vi "GTCP331-200ER - 1.C.(4).vi"(8 "error in (no error)":errorcluster, 11 "RT - Analysis Data in in in":T1={"Accel Sensistivity"=[0.0, 0.0, 0.0], "Cutoff Frequncies"=[{"LP Passband"=0.0, "HP Stopband"=0.0, "LP Stopband"=0.0, "HP Passband"=0.0}, {"LP Passband"=0.0, "HP Stopband"=0.0, "LP Stopband"=0.0, "HP Passband"=0.0}, {"LP Passband"=0.0, "HP Stopband"=0.0, "LP Stopband"=0.0, "HP Passband"=0.0}], "APU Setup File"={"Sensor Info"=[], "Calibration Info"=[], "CMM Table 106"=[], "CMM Table 106B "=[], "Accel Config"=[], "Report Sheet 1"=[], "Report Sheet 2"=[], "Report Sheet 3"=[]}, "RepairLevel"=""} {"Cutoff Frequncies"."HP Passband" min=1.0 step=1.0 format="%#.4f"; "Cutoff Frequncies"."LP Stopband" min=1.0 step=1.0 format="%#.4f"; "Cutoff Frequncies"."HP Stopband" min=1.0 step=1.0 format="%#.4f"; "Cutoff Frequncies"."LP Passband" min=1.0 step=1.0 format="%#.4f"}) -> (0 "error out":errorcluster, 2 "Interactive Mode Vals":dbl[](array[numeric]), 3 "RT - Analysis Data in out":T1 {"Cutoff Frequncies"."HP Passband" min=1.0 step=1.0 format="%#.4f"; "Cutoff Frequncies"."LP Stopband" min=1.0 step=1.0 format="%#.4f"; "Cutoff Frequncies"."HP Stopband" min=1.0 step=1.0 format="%#.4f"; "Cutoff Frequncies"."LP Passband" min=1.0 step=1.0 format="%#.4f"})   [LabVIEW 2018, in "RT - Analysis.lvlib"]
doc: "This subtest perfmors engine run-in procedures."
uses:
  RT - Analysis.lvlib
  Private Controls/Watchdog Settings.ctl
  Private Controls/Interactive Data.ctl
  <vilib>/Analysis/NI_AALBase.lvlib
  <vilib>/Analysis/baseanly.llb/Mean (DBL).vi
  Private Controls/RT-Analysis Data.ctl
  Modules/Testing UI 3/Private Controls/Cutoff Frequency.ctl
  Modules/Testing UI 3/Testing UI 3.lvlib
  Top Level/Shared Controls/APU Setup File.ctl
panel:
  # "Highpass Cutoff Frequency"
  # "Lowpass Cutoff Frequency"
  # "Highpass Cutoff Frequency"
  # "Lowpass Cutoff Frequency"
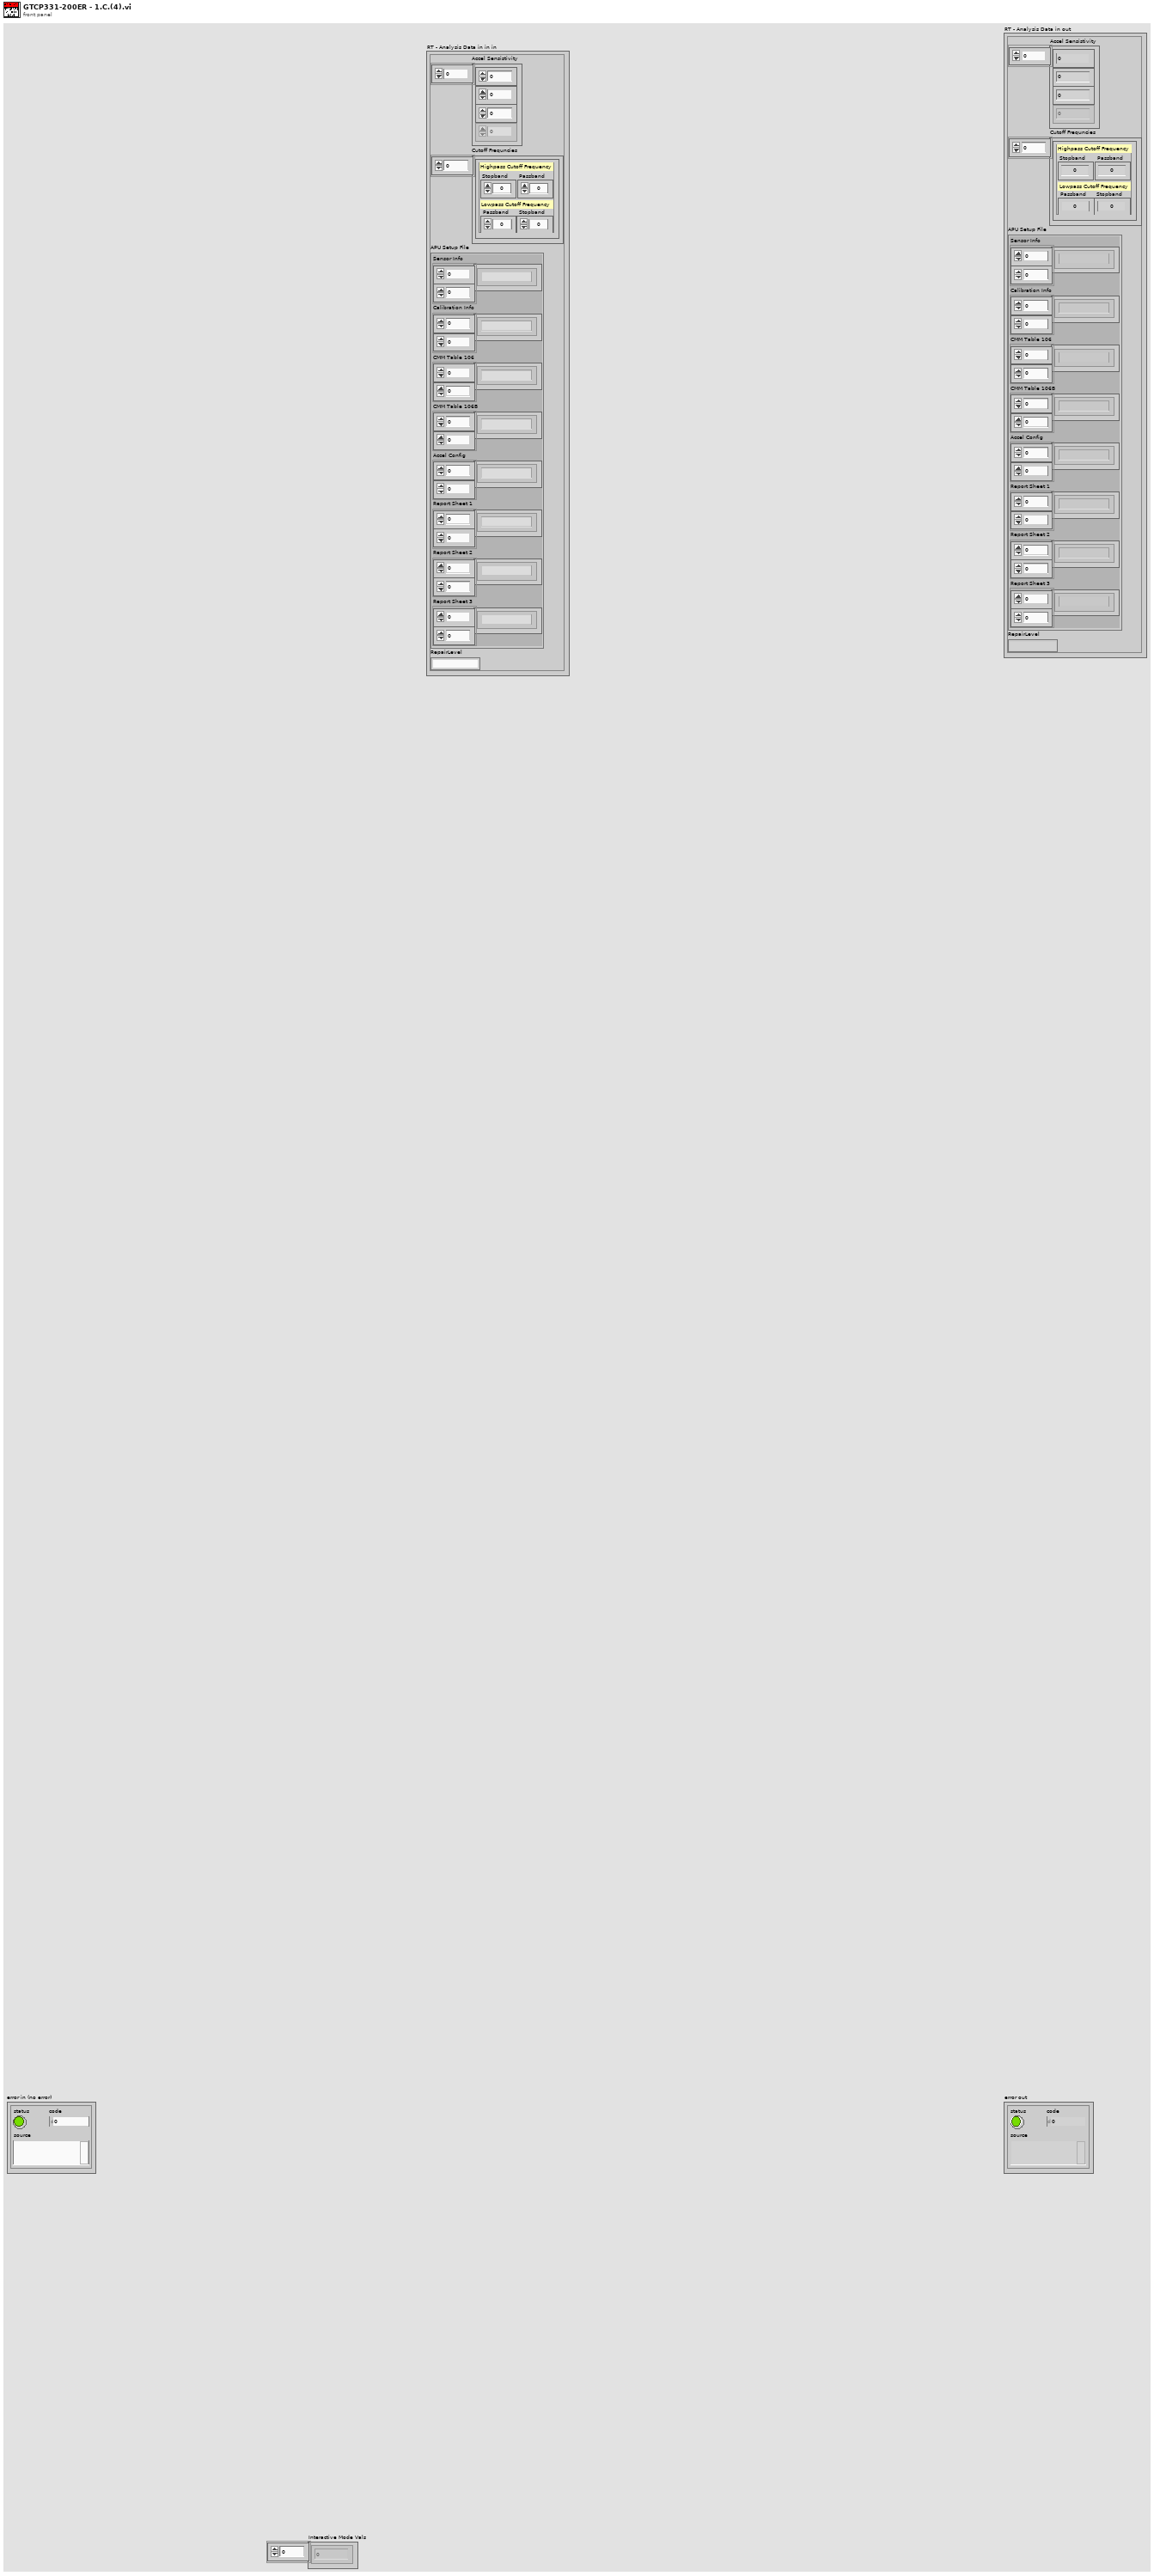
[diagram p1: front panel]
types:
  T1 = typedef "RT - Analysis.lvlib/RT-Analysis Data.ctl" = cluster{"Accel Sensistivity":dbl[], "Cutoff Frequncies":T2[], "APU Setup File":T3, "RepairLevel":string}
  T2 = typedef "Testing UI 3.lvlib/Cutoff Frequency.ctl" = cluster{"LP Passband":dbl, "HP Stopband":dbl, "LP Stopband":dbl, "HP Passband":dbl}
  T3 = typedef "APU Setup File.ctl" = cluster{"Sensor Info":string[][], "Calibration Info":string[][], "CMM Table 106":string[][], "CMM Table 106B ":string[][], "Accel Config":string[][], "Report Sheet 1":string[][], "Report Sheet 2":string[][], "Report Sheet 3":string[][]}
  T4 = typedef "RT - Analysis.lvlib/Watchdog Settings.ctl" = cluster{"Watchdog Action":enum16{"Disabled", "Timer - Change Sample Rate", "RPM Thresh - Insert Other", "RPM Thresh - Check POPD", "RPM Thresh - StartStop Logging"}, "Timer Start":timestamp, "[Watchdog Bools]":bool[], "[Watchdog DBLs]":dbl[], "Watchdog Variant":variant}
  T5 = typedef "RT - Analysis.lvlib/Interactive Data.ctl" = cluster{"Confirm Pressed":bool, "Stored Vals":dbl[]}
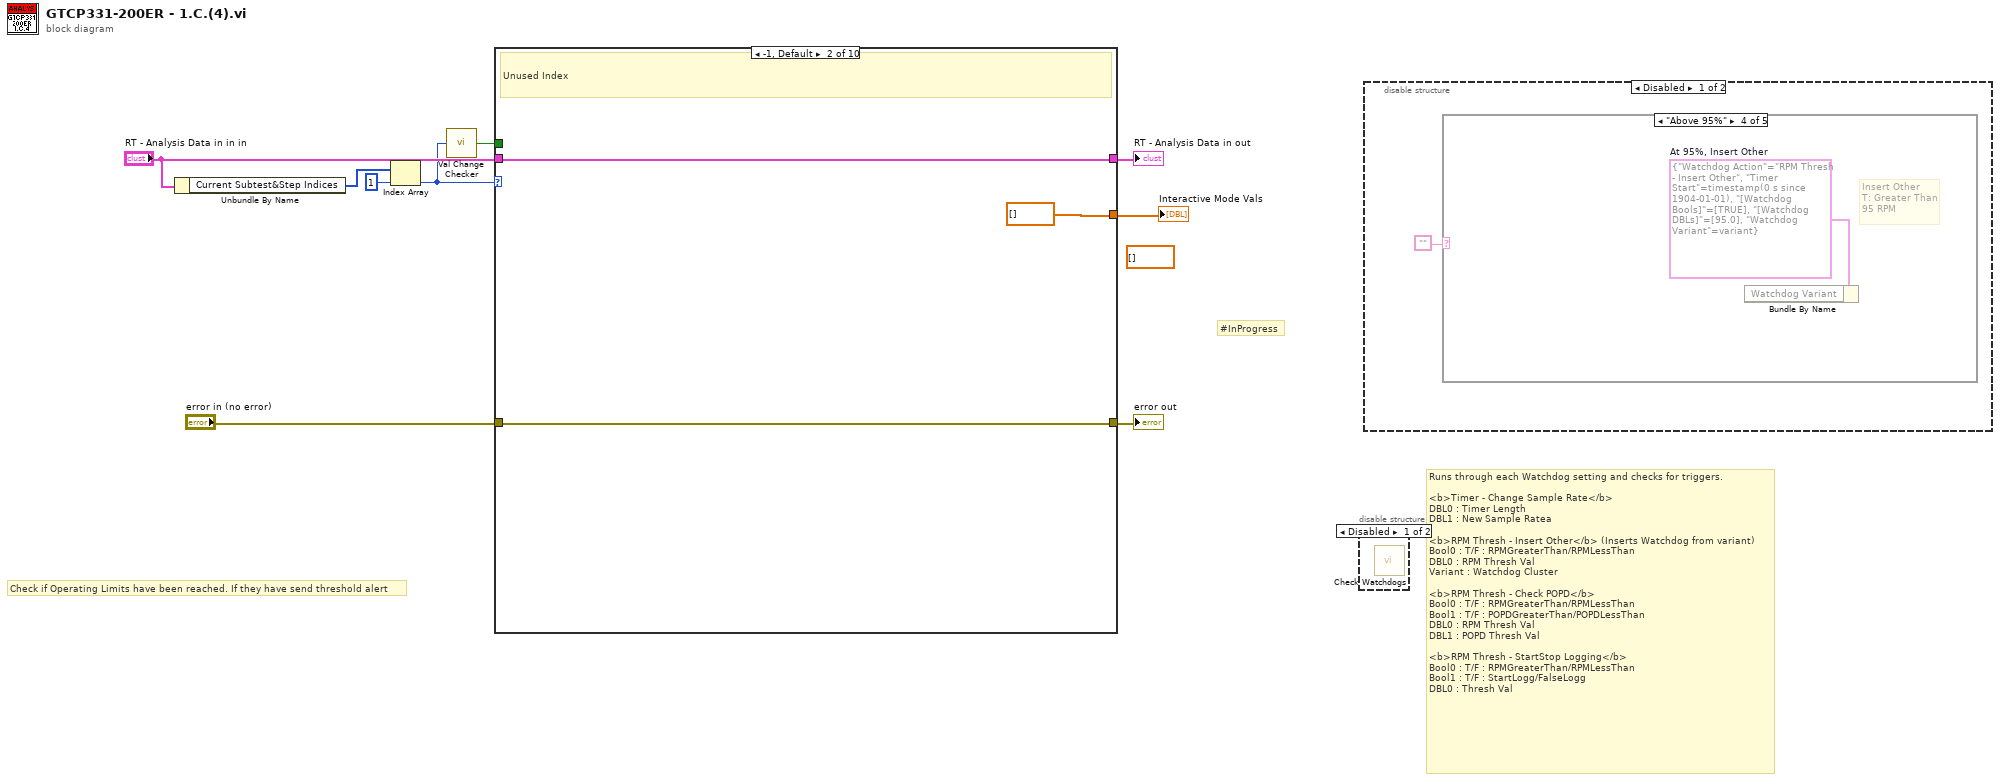
[diagram p0: block diagram]
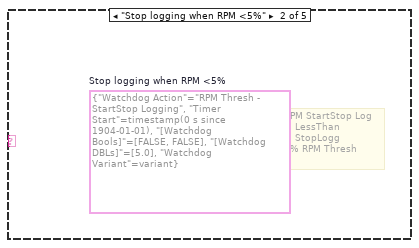
[diagram p3: hidden frame]
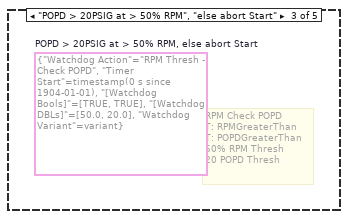
[diagram p4: hidden frame]
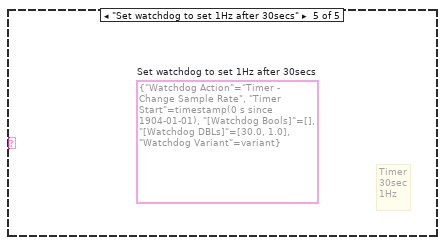
[diagram p5: hidden frame]
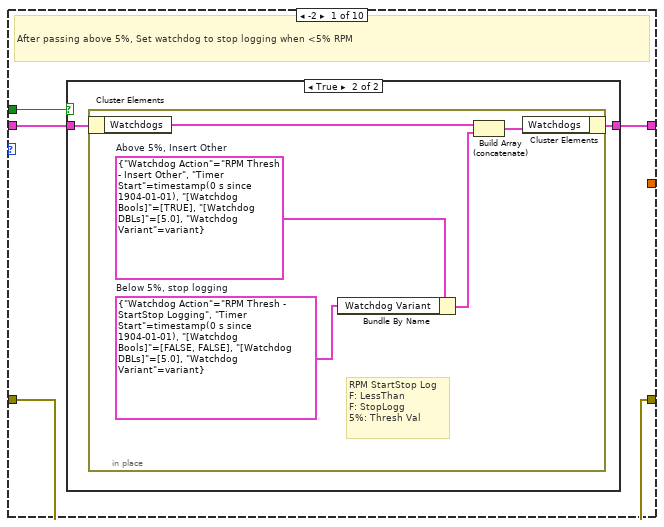
[diagram p8: hidden frame]
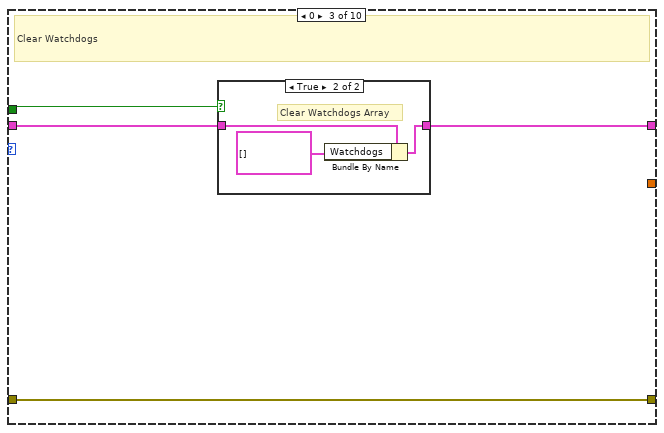
[diagram p10: hidden frame]
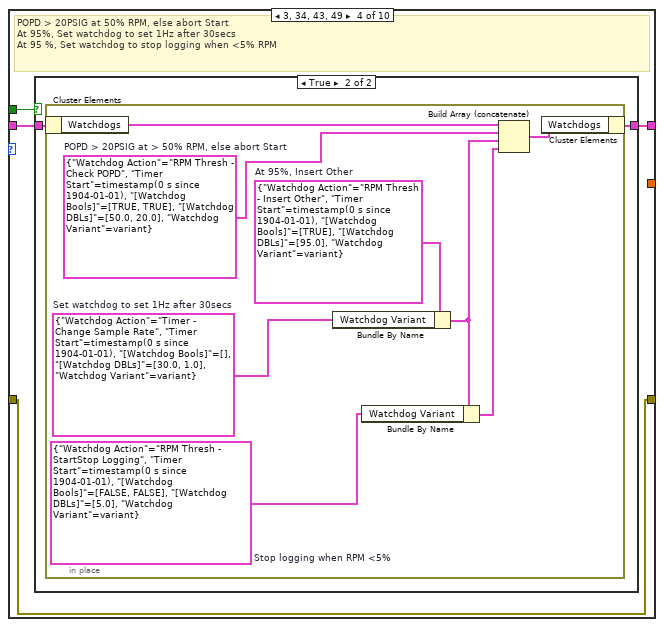
[diagram p12: hidden frame]
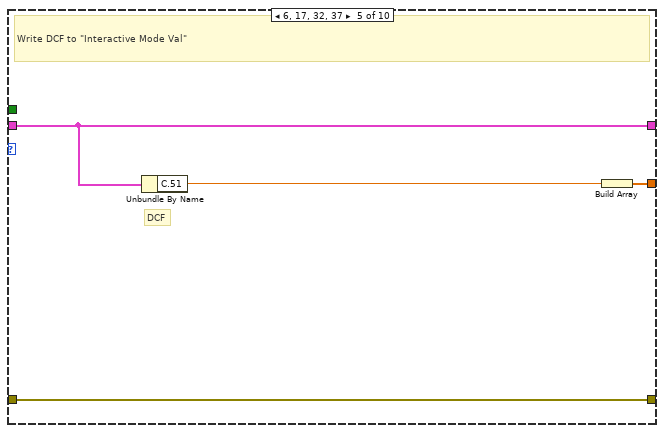
[diagram p14: hidden frame]
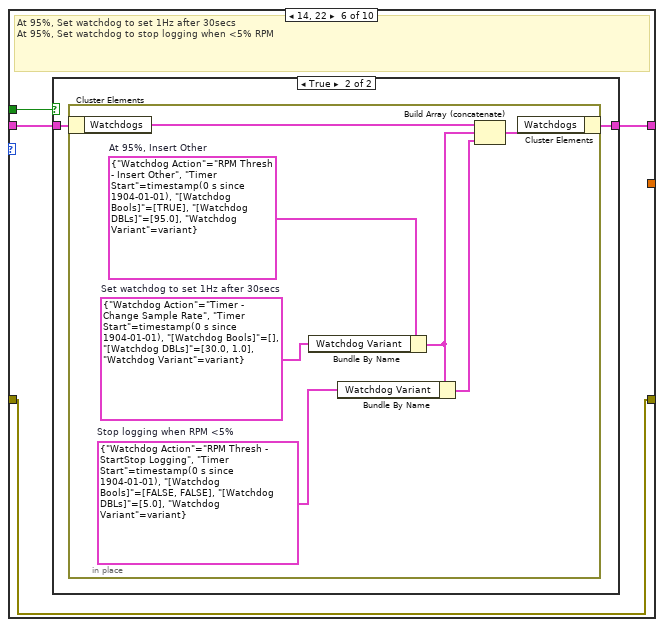
[diagram p15: hidden frame]
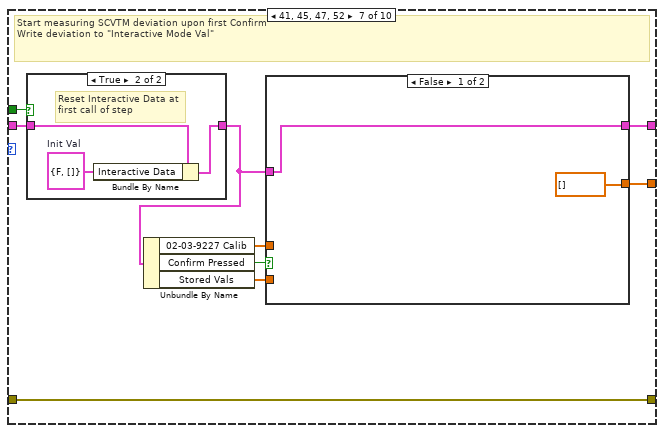
[diagram p17: hidden frame]
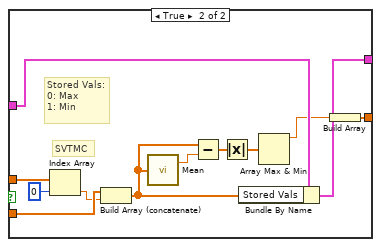
[diagram p18: hidden frame]
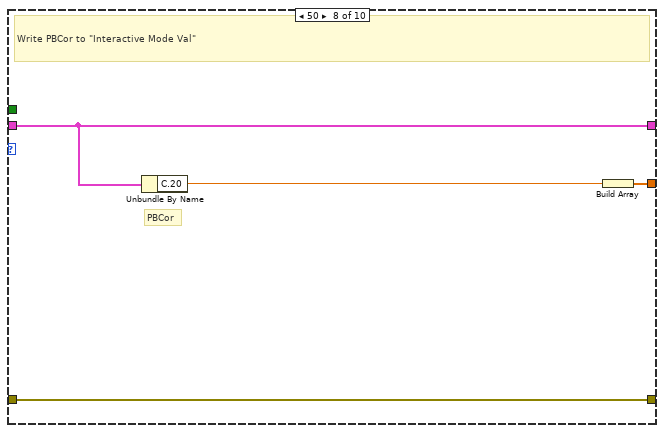
[diagram p20: hidden frame]
diagram:
  (unwired) dbl[] [] ("Interactive Mode Vals")
  # "#InProgress"
  # "Runs through each Watchdog setting and checks for triggers.\n\n<b>Timer - Change Sample Rate</b>\nDBL0 : Timer Length\nDBL1 : New Sample Ratea\n\n<b>RPM Thresh - Insert Other</b> (Inserts Watchdog from variant)\nBool0 : T/F : RPMGreaterThan/RPMLessThan\nDBL0 : RPM Thresh Val\nVariant : Watchdog Cluster\n\n<b>RPM Thresh - Check POPD</b>\nBool0 : T/F : RPMGreaterThan/RPMLessThan\nBool1 : T/F : POPDGreaterThan/POPDLessThan\nDBL0 : RPM Thresh Val\nDBL1 : POPD Thresh Val\n\n<b>RPM Thresh - StartStop Logging</b>\nBool0 : T/F : RPMGreaterThan/RPMLessThan\nBool1 : T/F : StartLogg/FalseLogg\nDBL0 : Thresh Val"
  # "Check if Operating Limits have been reached. If they have send threshold alert"
  n1 = Unbundle By Name("RT - Analysis Data in in in") -> ("Current Subtest&Step Indices"=w9:i32[])
  n2 = Index Array(array=w9, index=1) -> (element=w4:i32)
  n3 = call "Val Change Checker.vi"("Current Value in"=w4) -> ("Value Change?"=w3:bool)
  n4 = case shown="-1, Default" w4 {
    tunnel: [w13 w24 w28 w36 w51 w55 w74 w96 w100 w106] -> w7
    tunnel: "error in (no error)" -> [w13 w24 w28 w36 w51 w55 w74 w96 w100 w106]
    tunnel: [w12 w23 w26 w35 w50 w54 w67 w95 w99 w105] -> w6
    tunnel: "RT - Analysis Data in in in" -> [w11 w23 w27 w34 w50 w53 w71 w95 w99 w105]
    tunnel: [_ dbl[] [] ("Interactive Mode Vals") _ _ w48 _ w73 w93 w97 w104] -> w1
    tunnel: w3 -> [w10 _ w25 w33 _ w52 w72 _ _ _]
    frame -2 {
      # "After passing above 5%, Set watchdog to stop logging when <5% RPM"
      n5 = case shown="True" w10 {
        tunnel: [w14 w16] -> w12
        tunnel: w11 -> [w14 w15]
        frame False {
        }
        frame True {
          n6 = in-place {
            w17 = T4 {"Watchdog Action"=enum."RPM Thresh - StartStop Logging", "Timer Start"=timestamp(0 s since 1904-01-01), "[Watchdog Bools]"=[FALSE, FALSE], "[Watchdog DBLs]"=[5.0], "Watchdog Variant"=variant}  # Below 5%, stop logging
            w19 = T4 {"Watchdog Action"=enum."RPM Thresh - Insert Other", "Timer Start"=timestamp(0 s since 1904-01-01), "[Watchdog Bools]"=[TRUE], "[Watchdog DBLs]"=[5.0], "Watchdog Variant"=variant}  # Above 5%, Insert Other
            # "RPM StartStop Log\nF: LessThan\nF: StopLogg\n5%: Thresh Val"
            n7 = in-place-cluster #1(w15) -> ("Watchdogs"=w20:T4[])
            n8 = Bundle By Name(cluster=w19, "Watchdog Variant"=w17) -> (w18:T4)
            n9 = Build Array (concatenate)(w20, w18) -> (w21:T4[])
            n10 = in-place-cluster #1("Watchdogs"=w21) -> (w16:T1)
          }
        }
      }
    }
    frame -1, Default {
      # "Unused Index"
    }
    frame 0 {
      # "Clear Watchdogs"
      n11 = case shown="True" w25 {
        tunnel: w27 -> [w29 w32]
        tunnel: [w29 w31] -> w26
        frame False {
        }
        frame True {
          # "Clear Watchdogs Array"
          n12 = Bundle By Name(cluster=w32, "Watchdogs"=T4[] []) -> (w31:T1)
        }
      }
    }
    frame 3, 34, 43, 49 {
      # "POPD > 20PSIG at 50% RPM, else abort Start\nAt 95%, Set watchdog to set 1Hz after 30secs\nAt 95 %, Set watchdog to stop logging when <5% RPM"
      n13 = case shown="True" w33 {
        tunnel: [w37 w39] -> w35
        tunnel: w34 -> [w37 w38]
        frame False {
        }
        frame True {
          n14 = in-place {
            w40 = T4 {"Watchdog Action"=enum."RPM Thresh - StartStop Logging", "Timer Start"=timestamp(0 s since 1904-01-01), "[Watchdog Bools]"=[FALSE, FALSE], "[Watchdog DBLs]"=[5.0], "Watchdog Variant"=variant}  # Stop logging when RPM <5%
            w45 = T4 {"Watchdog Action"=enum."Timer - Change Sample Rate", "Timer Start"=timestamp(0 s since 1904-01-01), "[Watchdog Bools]"=[], "[Watchdog DBLs]"=[30.0, 1.0], "Watchdog Variant"=variant}  # Set watchdog to set 1Hz after 30secs
            w44 = T4 {"Watchdog Action"=enum."RPM Thresh - Insert Other", "Timer Start"=timestamp(0 s since 1904-01-01), "[Watchdog Bools]"=[TRUE], "[Watchdog DBLs]"=[95.0], "Watchdog Variant"=variant}  # At 95%, Insert Other
            w43 = T4 {"Watchdog Action"=enum."RPM Thresh - Check POPD", "Timer Start"=timestamp(0 s since 1904-01-01), "[Watchdog Bools]"=[TRUE, TRUE], "[Watchdog DBLs]"=[50.0, 20.0], "Watchdog Variant"=variant}  # POPD > 20PSIG at > 50% RPM, else abort Start
            n15 = in-place-cluster #2(w38) -> ("Watchdogs"=w46:T4[])
            n16 = Bundle By Name(cluster=w44, "Watchdog Variant"=w45) -> (w42:T4)
            n17 = Bundle By Name(cluster=w42, "Watchdog Variant"=w40) -> (w41:T4)
            n18 = Build Array (concatenate)(w46, w43, w42, w41) -> (w47:T4[])
            n19 = in-place-cluster #2("Watchdogs"=w47) -> (w39:T1)
          }
        }
      }
    }
    frame 6, 17, 32, 37 {
      # "DCF"
      # "Write DCF to \"Interactive Mode Val\""
      n20 = Unbundle By Name(w50) -> ("C.51"=w49:dbl)
      n21 = Build Array(w49) -> (w48:dbl[])
    }
    frame 14, 22 {
      # "At 95%, Set watchdog to set 1Hz after 30secs\nAt 95%, Set watchdog to stop logging when <5% RPM"
      n22 = case shown="True" w52 {
        tunnel: [w56 w58] -> w54
        tunnel: w53 -> [w56 w57]
        frame False {
        }
        frame True {
          n23 = in-place {
            w59 = T4 {"Watchdog Action"=enum."RPM Thresh - StartStop Logging", "Timer Start"=timestamp(0 s since 1904-01-01), "[Watchdog Bools]"=[FALSE, FALSE], "[Watchdog DBLs]"=[5.0], "Watchdog Variant"=variant}  # Stop logging when RPM <5%
            w63 = T4 {"Watchdog Action"=enum."Timer - Change Sample Rate", "Timer Start"=timestamp(0 s since 1904-01-01), "[Watchdog Bools]"=[], "[Watchdog DBLs]"=[30.0, 1.0], "Watchdog Variant"=variant}  # Set watchdog to set 1Hz after 30secs
            w62 = T4 {"Watchdog Action"=enum."RPM Thresh - Insert Other", "Timer Start"=timestamp(0 s since 1904-01-01), "[Watchdog Bools]"=[TRUE], "[Watchdog DBLs]"=[95.0], "Watchdog Variant"=variant}  # At 95%, Insert Other
            n24 = in-place-cluster #3(w57) -> ("Watchdogs"=w64:T4[])
            n25 = Bundle By Name(cluster=w62, "Watchdog Variant"=w63) -> (w61:T4)
            n26 = Bundle By Name(cluster=w61, "Watchdog Variant"=w59) -> (w60:T4)
            n27 = Build Array (concatenate)(w64, w61, w60) -> (w65:T4[])
            n28 = in-place-cluster #3("Watchdogs"=w65) -> (w58:T1)
          }
        }
      }
    }
    frame 41, 45, 47, 52 {
      # "Start measuring SCVTM deviation upon first Confirm\nWrite deviation to \"Interactive Mode Val\""
      n29 = case shown="True" w72 {
        tunnel: w71 -> [w89 w92]
        tunnel: [w89 w91] -> w70
        frame False {
        }
        frame True {
          w90 = T5 {"Confirm Pressed"=FALSE, "Stored Vals"=[]}  # Init Val
          # "Reset Interactive Data at\nfirst call of step"
          n30 = Bundle By Name(cluster=w92, "Interactive Data"=w90) -> (w91:T1)
        }
      }
      n31 = Unbundle By Name(w70) -> ("02-03-9227 Calib"=w66:dbl[], "Confirm Pressed"=w69:bool, "Stored Vals"=w68:dbl[])
      n32 = case shown="False" w69 {
        tunnel: [dbl[] [] ("Interactive Mode Vals") w77] -> w73
        tunnel: w70 -> [w76 w88]
        tunnel: w68 -> [_ w84]
        tunnel: [w76 w87] -> w67
        tunnel: w66 -> [_ w86]
        frame False {
        }
        frame True {
          # "Stored Vals:\n0: Max\n1: Min"
          # "SVTMC"
          n33 = Index Array(array=w86, index=0) -> (element=w83:dbl)
          n34 = Build Array (concatenate)(w84, w83) -> (w81:dbl[])
          n35 = call-poly <vilib>:"Mean.vi"("X"=w81) -> ("mean"=w82:dbl)  [unwired: 1 out]
          n36 = Subtract(x=w81, y=w82) -> (x-y=w80:dbl[])
          n37 = Absolute Value(x=w80) -> (abs(x)=w79:dbl[])
          n38 = Bundle By Name(cluster=w88, "Stored Vals"=w81) -> (w87:T1)
          n39 = Array Max & Min(array=w79) -> (max value=w78:dbl)  [unwired: 3 out]
          n40 = Build Array(w78) -> (w77:dbl[])
        }
      }
    }
    frame 50 {
      # "PBCor"
      # "Write PBCor to \"Interactive Mode Val\""
      n41 = Unbundle By Name(w95) -> ("C.20"=w94:dbl)
      n42 = Build Array(w94) -> (w93:dbl[])
    }
    frame 46 {
      # "PBCor"
      # "Write PBCor to \"Interactive Mode Val\""
      n43 = Unbundle By Name(w99) -> ("C.27"=w98:dbl)
      n44 = Build Array(w98) -> (w97:dbl[])
    }
    frame 44 {
      # "RPM 00-03-9402-00"
      # "Write PBCor to \"Interactive Mode Val\""
      n45 = Unbundle By Name(w105) -> ("00-03-9402 Calib"=w103:dbl[])
      n46 = Index Array(array=w103, index=0) -> (element=w101:dbl)
      n47 = Build Array(w101) -> (w104:dbl[])
    }
  }
  "RT - Analysis Data in out" <- w6
  "error out" <- w7
  "Interactive Mode Vals" <- w1
  n48 = disable-structure shown="Disabled" {
    frame Disabled {
      n49 = call "Check Watchdogs.vi"() -> ()  [unwired: 10 in, 2 out]
    }
    frame Enabled {
    }
  }
  n50 = disable-structure shown="Disabled" {
    frame Disabled {
      n51 = case shown="\"Above 95%\"" "" {
        frame Default {
        }
        frame "Stop logging when RPM <5%" {
          (unwired) T4 {"Watchdog Action"=enum."RPM Thresh - StartStop Logging", "Timer Start"=timestamp(0 s since 1904-01-01), "[Watchdog Bools]"=[FALSE, FALSE], "[Watchdog DBLs]"=[5.0], "Watchdog Variant"=variant}  # Stop logging when RPM <5%
          # "RPM StartStop Log\nF: LessThan\nF: StopLogg\n5% RPM Thresh"
        }
        frame "POPD > 20PSIG at > 50% RPM", "else abort Start" {
          (unwired) T4 {"Watchdog Action"=enum."RPM Thresh - Check POPD", "Timer Start"=timestamp(0 s since 1904-01-01), "[Watchdog Bools]"=[TRUE, TRUE], "[Watchdog DBLs]"=[50.0, 20.0], "Watchdog Variant"=variant}  # POPD > 20PSIG at > 50% RPM, else abort Start
          # "RPM Check POPD\nT: RPMGreaterThan\nT: POPDGreaterThan\n50% RPM Thresh\n20 POPD Thresh"
        }
        frame "Above 95%" {
          w108 = T4 {"Watchdog Action"=enum."RPM Thresh - Insert Other", "Timer Start"=timestamp(0 s since 1904-01-01), "[Watchdog Bools]"=[TRUE], "[Watchdog DBLs]"=[95.0], "Watchdog Variant"=variant}  # At 95%, Insert Other
          # "Insert Other\nT: Greater Than\n95 RPM"
          n52 = Bundle By Name(cluster=w108) -> ()  [unwired: 1 in, 1 out]
        }
        frame "Set watchdog to set 1Hz after 30secs" {
          (unwired) T4 {"Watchdog Action"=enum."Timer - Change Sample Rate", "Timer Start"=timestamp(0 s since 1904-01-01), "[Watchdog Bools]"=[], "[Watchdog DBLs]"=[30.0, 1.0], "Watchdog Variant"=variant}  # Set watchdog to set 1Hz after 30secs
          # "Timer\n30sec\n1Hz"
        }
      }
    }
    frame Enabled {
    }
  }
